vi "Set Setpoint.vi"(6 "parseError? T:Yes":bool=TRUE, 7 "Setpointindex (Setpoint1: Default)":enum16{"Setpoint 1", "Setpoint 2", "Setpoint 3"}(ring), 8 "error in (no error)":errorcluster, 10 "newSetpoint (20.00°C)":dbl=20.0, 11 "VISA resource name":refnum<visa-resource-name>) -> (0 "error out":errorcluster, 3 "VISA resource name out":refnum<visa-resource-name>)   [LabVIEW 2018, in "JULABO DeviceDriver.lvlib"]
doc: "This VI sends a new setpoint to the connected instrument. The adjustable setpoint range may range in dependence on the type of instrument and the adjusted limits. On using any value outside these limits an error occurs. The resolution is up to two digits (0.01 °C).\n\nNote:\nMost devices support up to three setpoints. Please note that the correct setpoint is selected for controlling."
uses:
  JULABO DeviceDriver.lvlib
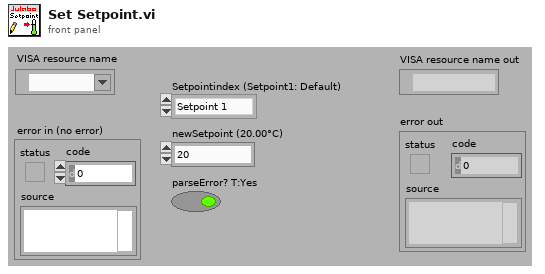
[diagram p1: front panel]
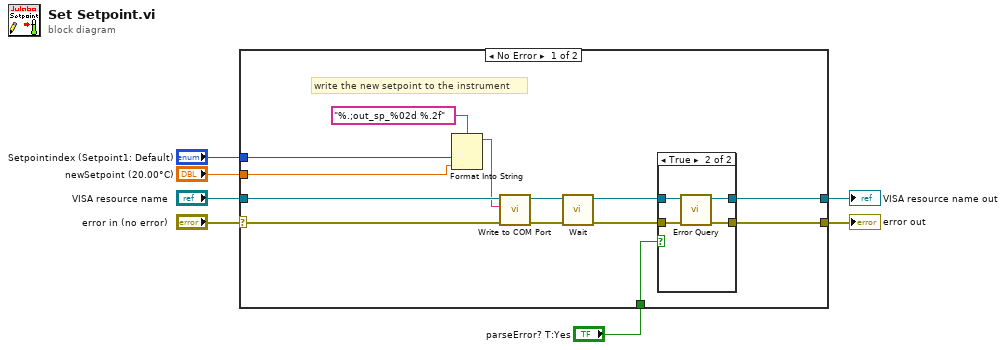
[diagram p0: block diagram]
diagram:
  n1 = case shown="No Error" "error in (no error)" {
    selector: "error in (no error)" -> [w19 w27]
    tunnel: "VISA resource name" -> [w20 w28]
    tunnel: [w17 w27] -> w6
    tunnel: [w16 w28] -> w5
    tunnel: "newSetpoint (20.00°C)" -> [w18 _]
    tunnel: "Setpointindex (Setpoint1: Default)" -> [w15 _]
    tunnel: "parseError? T:Yes" -> [w14 _]
    frame No Error {
      # "write the new setpoint to the instrument"
      n2 = Format Into String(format string="%.;out_sp_%02d %.2f", w15, w18) -> (resulting string=w12:string)  [unwired: 2 in, 1 out]
      n3 = call "Write to COM Port.vi"("error in"=w19, "Command (input)"=w12, "VISA resource name in"=w20) -> ("error out"=w10:errorcluster, "VISA resource name out"=w11:refnum<visa-resource-name>)  [unwired: 7 in]
      n4 = call "Wait.vi"("error in"=w10, "VISA resource name in"=w11) -> ("error out"=w8:errorcluster, "VISA resource name out"=w9:refnum<visa-resource-name>)  [unwired: 4 in]
      n5 = case shown="True" w14 {
        tunnel: w9 -> [w22 w26]
        tunnel: w8 -> [w21 w25]
        tunnel: [w22 w24] -> w16
        tunnel: [w21 w23] -> w17
        frame False {
        }
        frame True {
          n6 = call "Error Query.vi"("error in (no error)"=w25, "VISA resource name"=w26) -> ("error out"=w23:errorcluster, "VISA resource name out"=w24:refnum<visa-resource-name>)  [unwired: 6 in, 2 out]
        }
      }
    }
    frame Error {
    }
  }
  "error out" <- w6
  "VISA resource name out" <- w5
